vi "rqcBob Read PD State FIFO.vi"(8 "error in":errorcluster, 9 "timeout (ms)":i32=5000, 10 "number of elements":u32, 11 "FPGA reference in":refnum<k20>) -> (0 "error out":errorcluster, 1 "PM Level":u8[](array[numeric]), 2 "SPD Number":u8[](array[numeric]), 3 "FPGA reference out":refnum<k20>)   [LabVIEW 2018]
uses:
  <vilib>/Utility/error.llb/Error Cluster From Error Code.vi
  <vilib>/rvi/errors/niLvFpgaAdjustHostInterfaceError.vi
  <vilib>/rvi/interface/nirviMethod/nirviMethod.xnode
  <vilib>/rvi/errors/niLvFpgaMergeErrorWithErrorCode.vi
  <vilib>/FPGAPlugInAG/Dynamic/niLvFpga_ReadFifo_Dynamic.vi
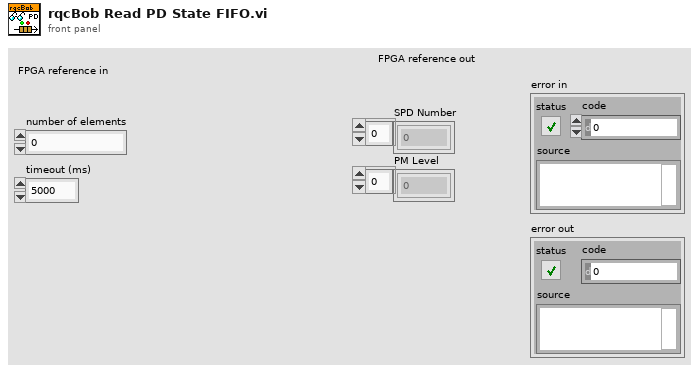
[diagram p1: front panel]
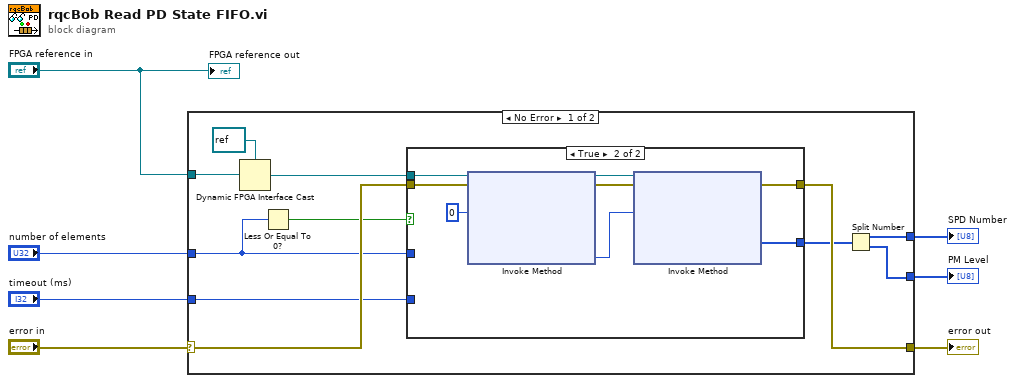
[diagram p0: block diagram]
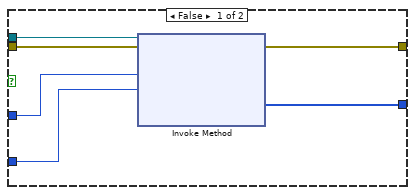
[diagram p2: hidden frame]
diagram:
  n1 = case shown="No Error" "error in" {
    selector: "error in" -> [w16 w33]
    tunnel: [w15 w33] -> w5
    tunnel: "FPGA reference in" -> [w18 _]
    tunnel: "number of elements" -> [w9 _]
    tunnel: "timeout (ms)" -> [w14 _]
    tunnel: [w12 _] -> w1
    tunnel: [w11 _] -> w2
    frame No Error {
      n2 = Dynamic FPGA Interface Cast(Session In=refnum<k20> refnum ("FPGA Interface"), Type=w18) -> (Session Out=w17:refnum<k20>)
      n3 = Less Or Equal To 0?(x=w9) -> (x <= 0?=w8:bool)
      n4 = case shown="True" w8 {
        tunnel: w9 -> [w22 _]
        tunnel: [w20 w30] -> w15
        tunnel: w17 -> [w24 w29]
        tunnel: w16 -> [w23 w28]
        tunnel: [w21 w25] -> w13
        tunnel: w14 -> [w19 _]
        frame False {
          n5 = xnode "Invoke Method"("FPGA VI Reference In"=w24, "error in"=w23, "Number of Elements"=w22, "Timeout (ms)"=w19) -> ("error out"=w20:errorcluster, "Data"=w21:u16[])  [unwired: 2 out]
        }
        frame True {
          n6 = xnode "Invoke Method"("FPGA VI Reference In"=w29, "error in"=w28, "Number of Elements"=u32 0) -> ("FPGA VI Reference Out"=w32:refnum<k20>, "error out"=w31:errorcluster, "Elements Remaining"=w27:u32)  [unwired: 1 in, 1 out]
          n7 = xnode "Invoke Method"("FPGA VI Reference In"=w32, "error in"=w31, "Number of Elements"=w27) -> ("error out"=w30:errorcluster, "Data"=w25:u16[])  [unwired: 1 in, 2 out]
        }
      }
      n8 = Split Number(x=w13) -> (hi(x)=w11:u8[], lo(x)=w12:u8[])
    }
    frame Error {
    }
  }
  "error out" <- w5
  "SPD Number" <- w2
  "PM Level" <- w1
  "FPGA reference out" <- "FPGA reference in"
